vi "Manual Assembly Temp.vi"() -> ()   [LabVIEW 2021]
uses:
  Classes/Assembly/Database Entry/Database Entry.lvclass
panel:
  out "Module":bool
  in  "Type":bool
  out "Status":dbl[][](array[numeric])
  in  "Assembly Region":T1
  in  "Stop":bool
  # "Protomodule"
  # "Module"
  # "Tray Slot 1"
  # "Slot 2"
  # "Slot 3"
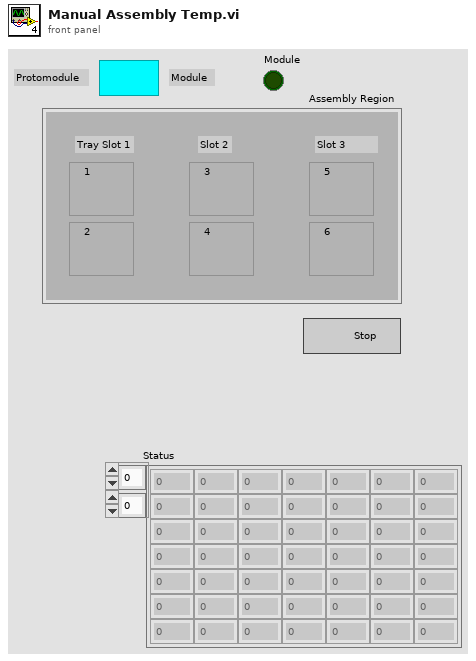
[diagram p1: front panel]
types:
  T1 = cluster{"1":bool, "2":bool, "3":bool, "4":bool, "5":bool, "6":bool}
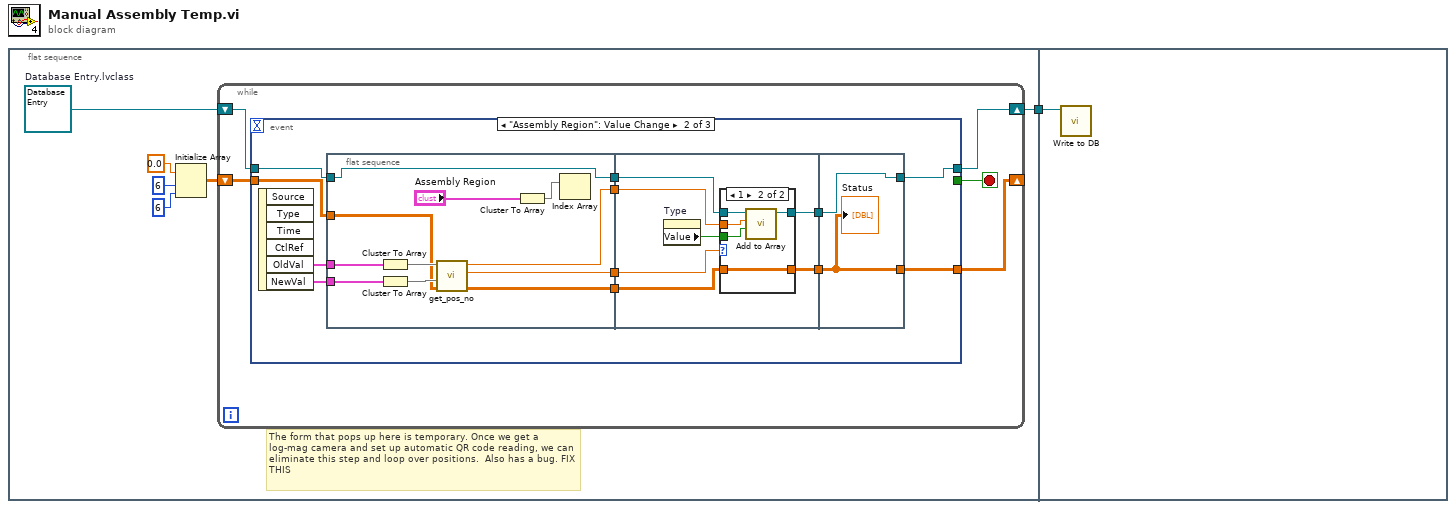
[diagram p0: block diagram]
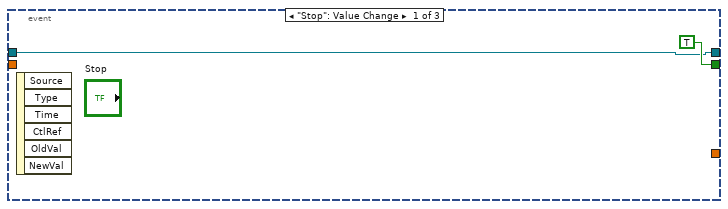
[diagram p2: hidden frame]
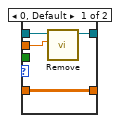
[diagram p3: hidden frame]
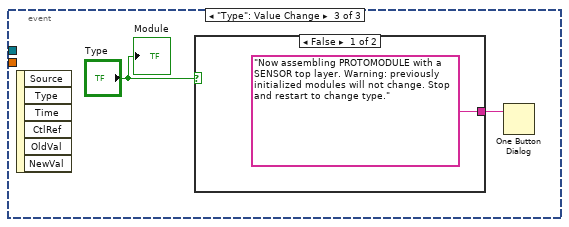
[diagram p4: hidden frame]
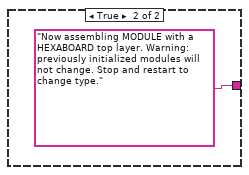
[diagram p5: hidden frame]
diagram:
  n1 = flat-sequence {
    tunnel: [w2] -> w1
    tunnel: w1 -> [w60]
    frame #0 {
      w3 = refnum<class "Database Entry.lvclass"> refnum  # Database Entry.lvclass
      # "The form that pops up here is temporary. Once we get a log-mag camera and set up automatic QR code reading, we can eliminate this step and loop over positions.  Also has a bug. FIX THIS"
      n2 = Initialize Array(0.0 ("element"), 6 ("dimension size"), 6 ("dimension size")) -> (w4:dbl[][])
      n3 = while {
        shift-right: [w11] -> w2
        shift-left: w3 -> [w8]
        shift-right: [w9] -> _
        shift-left: w4 -> [w10]
        stop <- w12 stop-if-true
        n4 = event shown="[1] \"Assembly Region\": Value Change" {
          selector: _ -> [_ _ _]
          dyn-events: _ -> [_ _ _]
          timeout: _ -> [_ _ _]
          tunnel: [TRUE _ _] -> w12
          tunnel: w8 -> [w13 w19 _]
          tunnel: [w13 w16 _] -> w11
          tunnel: w10 -> [_ w24 _]
          tunnel: [_ w20 _] -> w9
          event "Stop": Value Change {
            n5 = event-data() -> ()  [unwired: 1 in, 6 out]
          }
          event "Assembly Region": Value Change {
            n6 = event-data() -> ("OldVal"=w25:T1, "NewVal"=w26:T1)  [unwired: 1 in, 4 out]
            n7 = flat-sequence {
              tunnel: w26 -> [w36]
              tunnel: w25 -> [w35]
              tunnel: w24 -> [w31]
              tunnel: [w28] -> w22
              tunnel: [w30] -> w21
              tunnel: w19 -> [w29]
              tunnel: [w29] -> w18
              tunnel: [w27] -> w17
              tunnel: [w43] -> w23
              tunnel: w22 -> [w44]
              tunnel: w21 -> [w41]
              tunnel: w18 -> [w42]
              tunnel: w17 -> [w40]
              tunnel: [w39] -> w15
              tunnel: w23 -> [w55]
              tunnel: [w55] -> w20
              tunnel: [w54] -> w16
              tunnel: w15 -> [w54]
              frame #0 {
                n8 = Cluster To Array(cluster=w35) -> (array=w32:bool[])
                n9 = Cluster To Array(cluster=w36) -> (array=w33:bool[])
                n10 = call "get_pos_no.vi"("Status Old"=w31, "Array New Status"=w33, "Array Old Status"=w32) -> ("Status New"=w28:dbl[][], "State"=w27:dbl, "Position ID"=w30:dbl)  [unwired: 2 in]
                n11 = Cluster To Array(cluster="Assembly Region") -> (array=w37:bool[])
                n12 = Index Array(array=w37) -> ()  [unwired: 1 in, 1 out]
              }
              frame #1 {
                n13 = property on="Type" class="Bool (strict)"() -> ("Value"=w38:bool)  [unwired: 2 in, 2 out]
                n14 = case shown="1" w40 {
                  tunnel: w44 -> [w45 w53]
                  tunnel: [w45 w53] -> w43
                  tunnel: w42 -> [w48 w52]
                  tunnel: [w47 w51] -> w39
                  tunnel: w41 -> [w46 w50]
                  tunnel: w38 -> [_ w49]
                  frame 0, Default {
                    n15 = call "Remove.vi"("Index"=w46, "Database Entry in"=w48) -> ("Database Entry out"=w47:refnum<class "Database Entry.lvclass">)  [unwired: 8 in, 1 out]
                  }
                  frame 1 {
                    n16 = call "Add to Array.vi"("Module?"=w49, "Position Index"=w50, "Database Entry in"=w52) -> ("Database Entry out"=w51:refnum<class "Database Entry.lvclass">)  [unwired: 7 in, 1 out]
                  }
                }
              }
              frame #2 {
                "Status" <- w55
              }
            }
          }
          event "Type": Value Change {
            n17 = event-data() -> ()  [unwired: 1 in, 6 out]
            n18 = case shown="False" "Type" {
              tunnel: ["Now assembling PROTOMODULE with a SENSOR top layer. Warning: previously initialized modules will not change. Stop and restart to change type." "Now assembling MODULE with a HEXABOARD top layer. Warning: previously initialized modules will not change. Stop and restart to change type."] -> w57
              frame False {
              }
              frame True {
              }
            }
            n19 = One Button Dialog(message=w57) -> ()  [unwired: 1 in, 1 out]
            "Module" <- "Type"
          }
        }
      }
    }
    frame #1 {
      n20 = call "Write to DB.vi"("Database Entry in"=w60) -> ()  [unwired: 9 in, 2 out]
    }
  }
